vi "View Trend Graph.vi"() -> ()   [LabVIEW 2021]
panel:
  out "Current Value":dbl[](array[numeric])
  in  "stop":bool
  in  "file path (use dialog)":path=path "C:/Users/manma/Google Drive/WPC Stat Scrape/Data/WPC Stats.bin"
  in  "Trend Plot to View":T1(ring)=enum."Total Profit"
  out "XY Graph":cluster{timestamp[], dbl[]}[](graph)
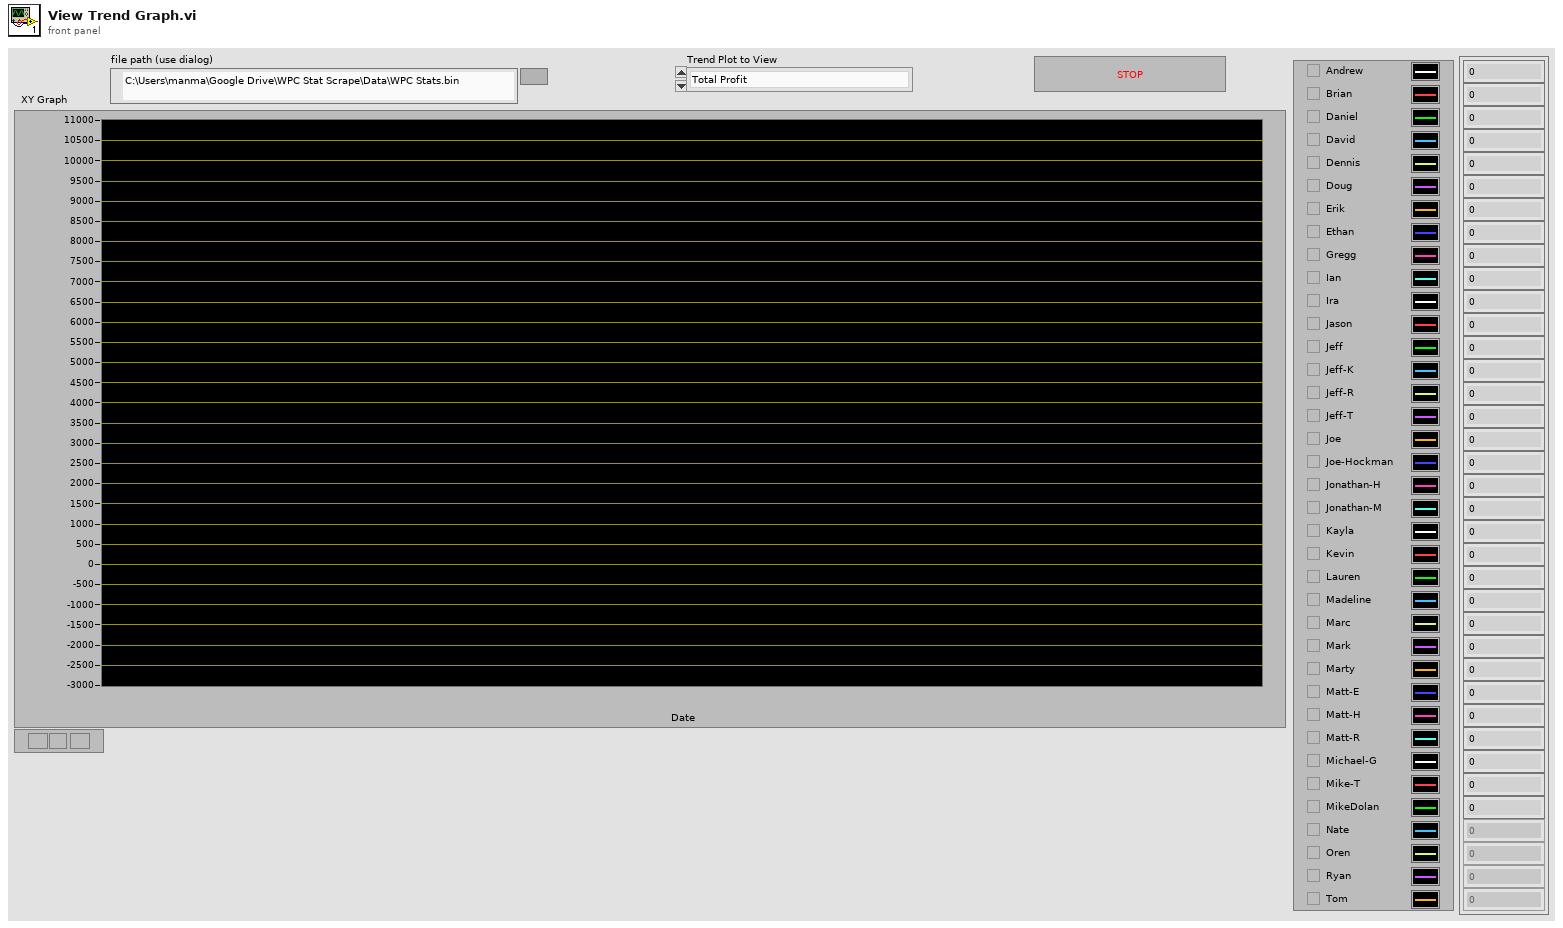
[diagram p1: front panel]
types:
  T1 = enum16{"Tournament Hands Played %", "Tournament Hands Won %", "Tournament Average Hands Dealt", "Tournament Average Hands Won", "Cash Hands Played %", "Cash Hands Won %", "Tournament Profit", "Cash Profit", "Total Profit", "Cash ROI", "Tournament ROI"}
  T2 = typedef "WPC Player and Financial Stats.ctl" = cluster{"Player Name":string, "Date Updated":timestamp, "Tournament Stats":cluster{"Hands Won":i32, "Hands Played":i32, "Hands Dealt":i32, "All-Ins":i32, "Entered":i32, "Winnings":dbl, "Profit":dbl}, "Cash Stats":cluster{"Hands Won":i32, "Hands Played":i32, "Hands Dealt":i32, "All-Ins":i32, "Profit":dbl}}
  T3 = cluster{"Hands Won":i32, "Hands Played":i32, "Hands Dealt":i32, "All-Ins":i32, "Entered":i32, "Winnings":dbl, "Profit":dbl}
  T4 = cluster{"Hands Won":i32, "Hands Played":i32, "Hands Dealt":i32, "All-Ins":i32, "Profit":dbl}
  T5 = cluster{"Hands Played %":dbl, "Hands Won %":dbl, "Average Hands Dealt Per Tournament":dbl, "Average Hands Won Per Tournament":dbl, "Average Hands Played Per Tournament":dbl, "Average All-Ins Per Tournament":dbl, "Average Winnings per Tournament":dbl, "Average Profit per Tournament":dbl}
  T6 = cluster{"Hands Played %":dbl, "Hands Won %":dbl, "All-In %":dbl, "Profit per Hand":dbl}
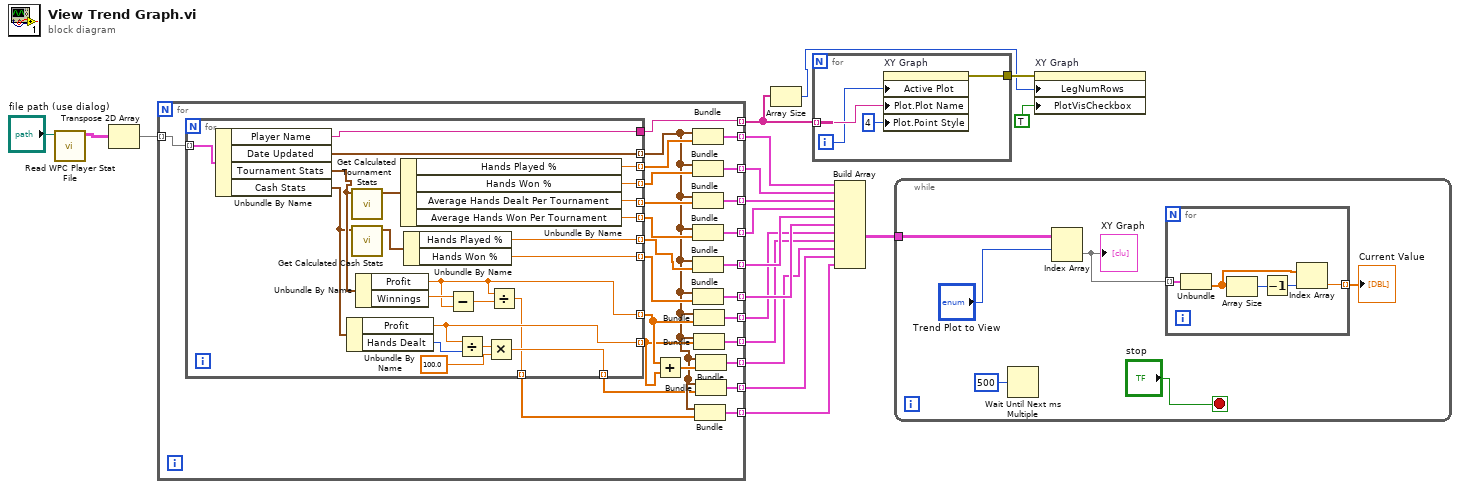
[diagram p0: block diagram]
diagram:
  n1 = call "Read WPC Player Stat File.vi"("file path (use dialog)"="file path (use dialog)") -> ("Full WPC Stats"=w10:T2[][])  [unwired: 8 in, 2 out]
  n2 = Transpose 2D Array(2D array=w10) -> (transposed array=w19:T2[][])
  n3 = for {
    tunnel: w19 -> [w44] mode=indexing
    tunnel: [w41] -> w11 mode=indexing
    tunnel: [w40] -> w18 mode=indexing
    tunnel: [w39] -> w17 mode=indexing
    tunnel: [w38] -> w16 mode=indexing
    tunnel: [w37] -> w15 mode=indexing
    tunnel: [w36] -> w14 mode=indexing
    tunnel: [w35] -> w13 mode=indexing
    tunnel: [w27] -> w5 mode=indexing
    tunnel: [w26] -> w4 mode=indexing
    tunnel: [w23] -> w3 mode=indexing
    tunnel: [w22] -> w2 mode=indexing
    tunnel: [w20] -> w1 mode=indexing
    n4 = for {
      tunnel: w44 -> [w66] mode=indexing
      tunnel: [w63] -> w41
      tunnel: [w62] -> w25 mode=indexing
      tunnel: [w61] -> w33 mode=indexing
      tunnel: [w60] -> w34 mode=indexing
      tunnel: [w59] -> w43 mode=indexing
      tunnel: [w58] -> w42 mode=indexing
      tunnel: [w57] -> w31 mode=indexing
      tunnel: [w56] -> w32 mode=indexing
      tunnel: [w48] -> w30 mode=indexing
      tunnel: [w54] -> w29 mode=indexing
      tunnel: [w51] -> w24 mode=indexing
      tunnel: [w47] -> w21 mode=indexing
      n5 = Unbundle By Name(w66) -> ("Player Name"=w63:string, "Date Updated"=w62:timestamp, "Tournament Stats"=w55:T3, "Cash Stats"=w45:T4)
      n6 = Unbundle By Name(w45) -> ("Profit"=w54:dbl, "Hands Dealt"=w46:i32)
      n7 = call "Get Calculated Tournament Stats.vi"("Tournament Stats"=w55) -> ("Calculated Tournament Stats"=w65:T5)  [unwired: 10 in]
      n8 = call "Get Calculated Cash Stats.vi"("Cash Stats"=w45) -> ("Calculated Cash Stats"=w64:T6)  [unwired: 10 in]
      n9 = Unbundle By Name(w55) -> ("Profit"=w48:dbl, "Winnings"=w50:dbl)
      n10 = Unbundle By Name(w65) -> ("Hands Played %"=w61:dbl, "Hands Won %"=w60:dbl, "Average Hands Dealt Per Tournament"=w59:dbl, "Average Hands Won Per Tournament"=w58:dbl)
      n11 = Unbundle By Name(w64) -> ("Hands Played %"=w57:dbl, "Hands Won %"=w56:dbl)
      n12 = Subtract(x=w50, y=w48) -> (x-y=w49:dbl)
      n13 = Divide(x=w54, y=w46) -> (x/y=w53:dbl)
      n14 = Multiply(x=w53, y=100.0) -> (x*y=w51:dbl)
      n15 = Divide(x=w48, y=w49) -> (x/y=w47:dbl)
    }
    n16 = Add(x=w30, y=w29) -> (x+y=w28:dbl[])
    n17 = Bundle(w25, w33) -> (w40:cluster{timestamp[], dbl[]})  [unwired: 1 in]
    n18 = Bundle(w25, w34) -> (w39:cluster{timestamp[], dbl[]})  [unwired: 1 in]
    n19 = Bundle(w25, w43) -> (w38:cluster{timestamp[], dbl[]})  [unwired: 1 in]
    n20 = Bundle(w25, w42) -> (w37:cluster{timestamp[], dbl[]})  [unwired: 1 in]
    n21 = Bundle(w25, w31) -> (w36:cluster{timestamp[], dbl[]})  [unwired: 1 in]
    n22 = Bundle(w25, w32) -> (w35:cluster{timestamp[], dbl[]})  [unwired: 1 in]
    n23 = Bundle(w25, w30) -> (w27:cluster{timestamp[], dbl[]})  [unwired: 1 in]
    n24 = Bundle(w25, w29) -> (w26:cluster{timestamp[], dbl[]})  [unwired: 1 in]
    n25 = Bundle(w25, w21) -> (w20:cluster{timestamp[], dbl[]})  [unwired: 1 in]
    n26 = Bundle(w25, w28) -> (w23:cluster{timestamp[], dbl[]})  [unwired: 1 in]
    n27 = Bundle(w25, w24) -> (w22:cluster{timestamp[], dbl[]})  [unwired: 1 in]
  }
  n28 = Array Size(array=w11) -> (size(s)=w8:i32)
  n29 = for {
    tunnel: w11 -> [w70] mode=indexing
    tunnel: [w68] -> w9
    i -> [w69]
    n30 = property on="XY Graph" class="XYGraph (strict)"("Active Plot"=w69, "Plot.Plot Name"=w70, "Plot.Point Style"=u8 4) -> (error out=w68:errorcluster)  [unwired: 2 in, 1 out]
  }
  n31 = Build Array(w18, w17, w16, w15, w14, w13, w5, w4, w3, w2, w1) -> (w12:cluster{timestamp[], dbl[]}[][])
  n32 = while {
    tunnel: w12 -> [w76]
    stop <- "stop" stop-if-true
    n33 = Wait Until Next ms Multiple(millisecond multiple=u32 500) -> ()  [unwired: 1 out]
    n34 = Index Array(array=w76, index (row)="Trend Plot to View") -> (element=w72:cluster{timestamp[], dbl[]}[])  [unwired: 1 in]
    "XY Graph" <- w72
    n35 = for {
      tunnel: w72 -> [w81] mode=indexing
      tunnel: [w77] -> w71 mode=indexing
      n36 = Unbundle(w81) -> (w78:dbl[])  [unwired: 1 out]
      n37 = Array Size(array=w78) -> (size(s)=w80:i32)
      n38 = Decrement(x=w80) -> (x-1=w79:i32)
      n39 = Index Array(array=w78, index=w79) -> (element=w77:dbl)
    }
    "Current Value" <- w71
  }
  n40 = property on="XY Graph" class="XYGraph (strict)"(error in=w9, "LegNumRows"=w8, "PlotVisCheckbox"=TRUE ("Legend:Plot Visibility Checkbox Visible")) -> ()  [unwired: 1 in, 2 out]
